vi "CPP-5168-PressureAnalysis-2012.vi"() -> (5 "Plug in titles":string[](array[string]), 7 "Plug in values":string[](array[string]))   [LabVIEW 2012]
uses:
  Globals/Meas_global.vi
  <vilib>/Analysis/baseanly.llb/Mean (DBL).vi
  <vilib>/measure/mascope.llb/Transition Measurements 1 chan.vi
  <vilib>/measure/NI_MAPro.lvlib
  <vilib>/Analysis/NI_AALBase.lvlib
panel:
  out "ValveShutAt":dbl format="%.2f"
  out "SourceOffIndex":i32
  out "nOpen":i32
  out "Zeroes?":bool
  out "Zeroes":dbl[](array[numeric])
  out "Data":dbl[][](array[numeric]) caption="ZeroedCompensatedCalibratedData" format="%#_3g"
  out "ChannelNames":string[](array[string])
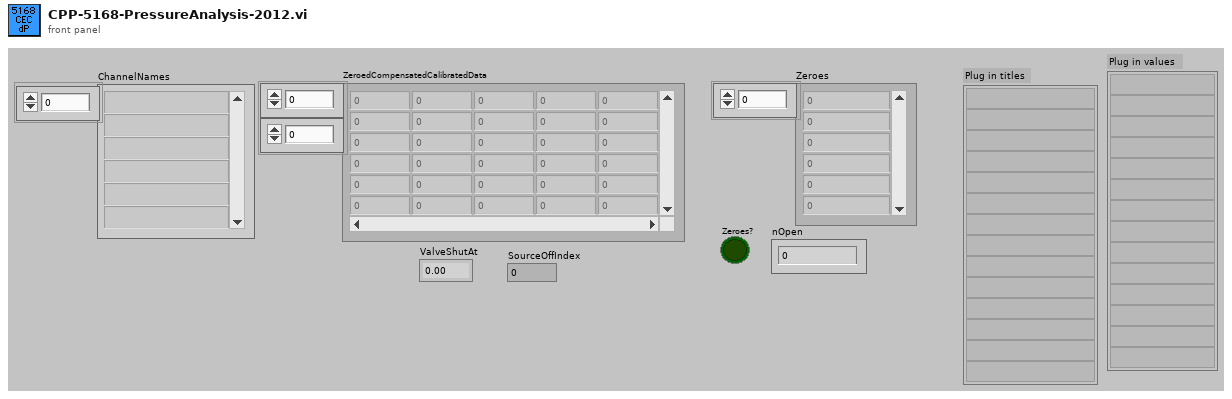
[diagram p1: front panel]
types:
  T1 = typedef "Analysis_info_cluster.ctl" = cluster{"Colour":u32, "Inst type":T2, "Inst name":string, "Symbol":string, "Code name":string, "Extra Info":string, "Inst Array":T3, "Extra Titles":string[], "Extra Values":string[], "U":dbl, "u^2":dbl, "u^3":dbl, "u^4":dbl, "Skew_u":dbl, "Kurt_u":dbl, "Sd Error in Mean":dbl, "% u'/U":dbl, "X":dbl, "Y":dbl, "Z":dbl, "Timescale integral to 25%":dbl, "Sd Error in Variance":dbl, "Calib File":path, "Calib Constants":dbl[], "Output Position":bool, "Full Stats":bool, "Av Sampling Rate":dbl, "Av No of Samples":dbl, "Total Meas Time (s)":dbl, "ADAM Ch Name":string}
  T2 = typedef "Inst_type.ctl" = enum16{"Propeller anemometer", "Raw voltage", "Pressure Transducer", "Pitot-static tube", "Preston tube", "Hot wire", "Cross wire 1", "Cross wire 2", "Generic Linear", "Generic Polynomial", "Generic BackPoly", "Fast FID", "Thermocouple", "Cold wire", "Pulsed Wire", "LDA Vel", "LDA Tran time", "LDA Arr time"}
  T3 = typedef "Instrument_Array.ctl" = enum16{"PWA", "LDA", "Analogue"}
  T4 = typedef "Time_Trace_Cluster.ctl" = cluster{"Weighting":dbl[], "Time (s)":dbl[], "Voltage":dbl[], "Eng Values":dbl[]}
  T5 = cluster{"start time":dbl, "end time":dbl, "ref levels":cluster{"high ref level":dbl, "mid ref level":dbl, "low ref level":dbl, "ref units":u16}}
  T6 = typedef "WindowDescriptor.ctl" = cluster{"Window\nName":string, "SurroundingTaps":string[], "TapWeights":dbl[], "OpenArea\nmm^2":dbl, "OpenArea\nFraction":dbl}
  T7 = typedef "WindowTimeseriesCluster.ctl" = cluster{"Name":string, "OpenArea(mm^2)":dbl, "Timeseries":dbl[]}
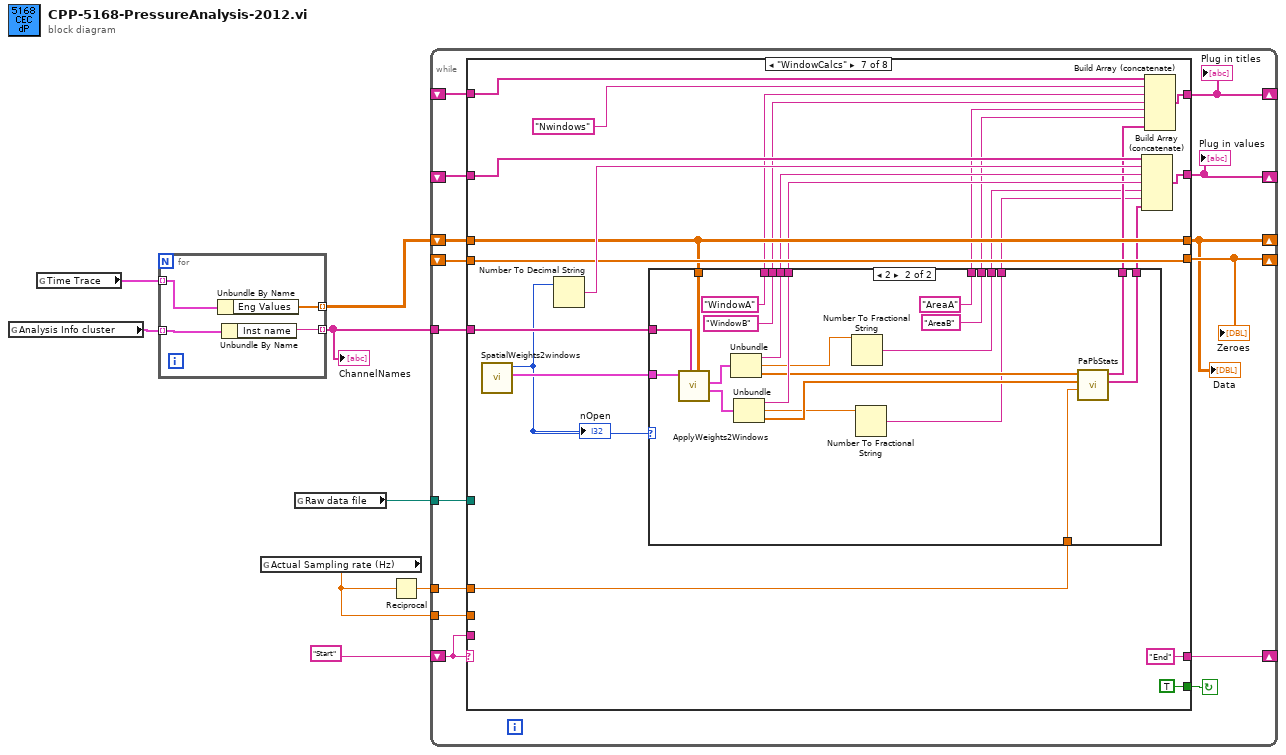
[diagram p0: block diagram]
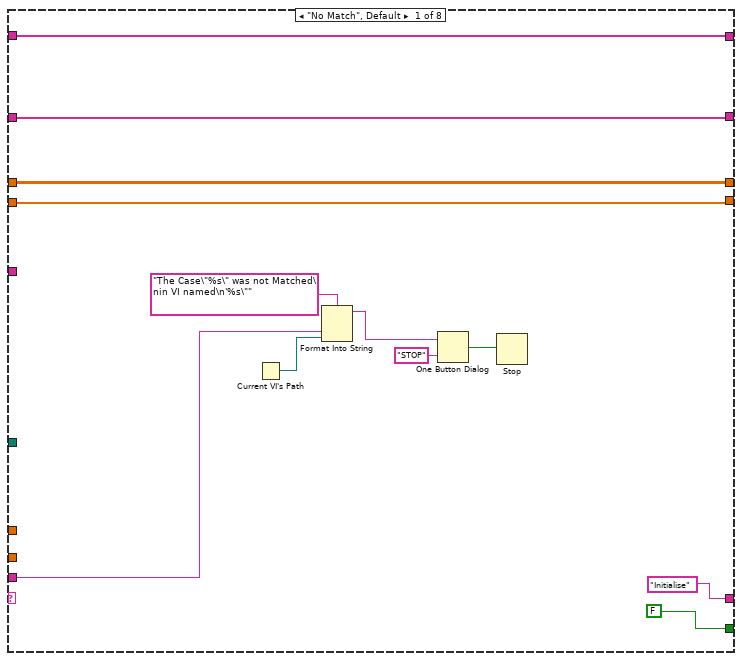
[diagram p2: hidden frame]
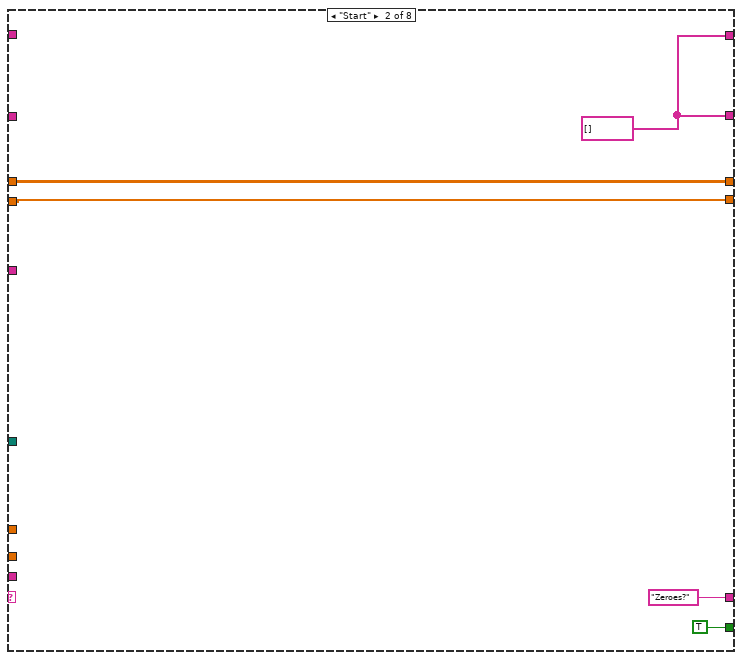
[diagram p3: hidden frame]
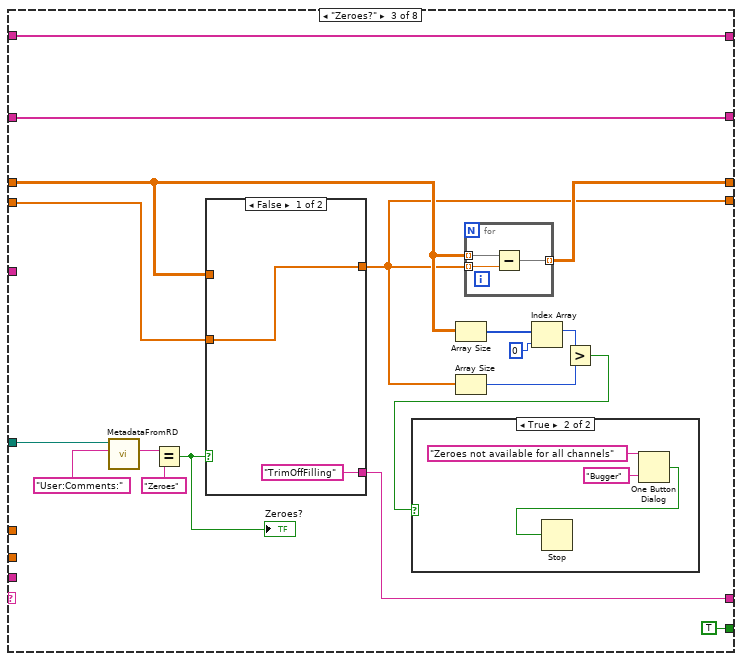
[diagram p4: hidden frame]
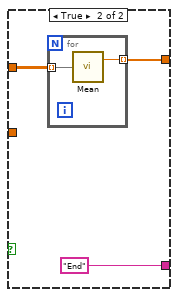
[diagram p6: hidden frame]
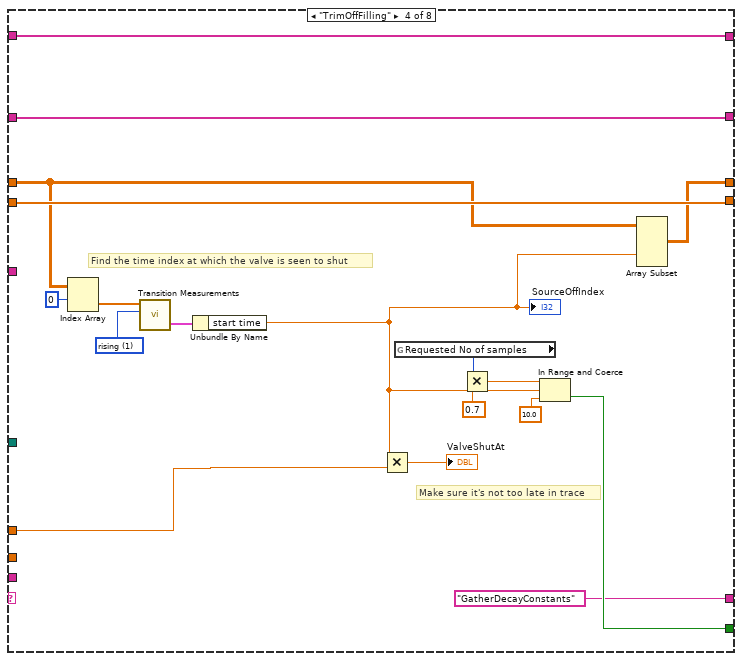
[diagram p7: hidden frame]
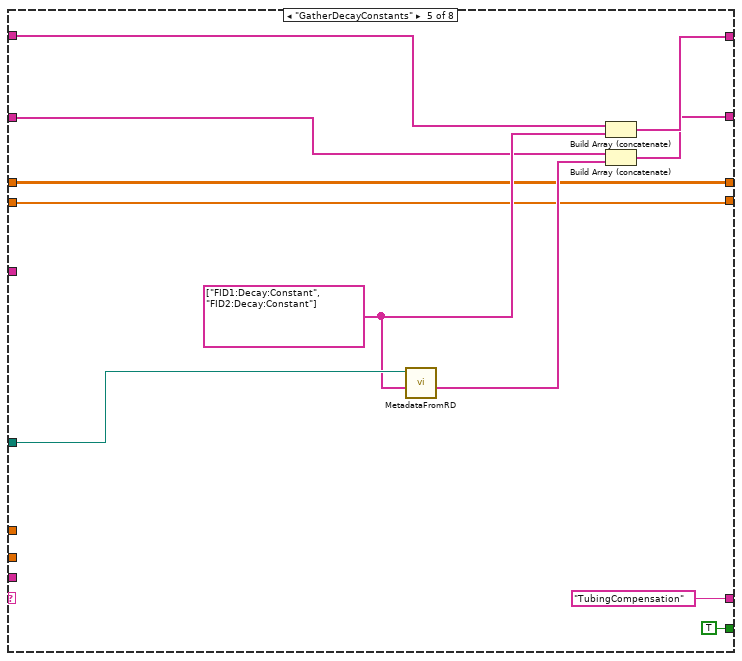
[diagram p8: hidden frame]
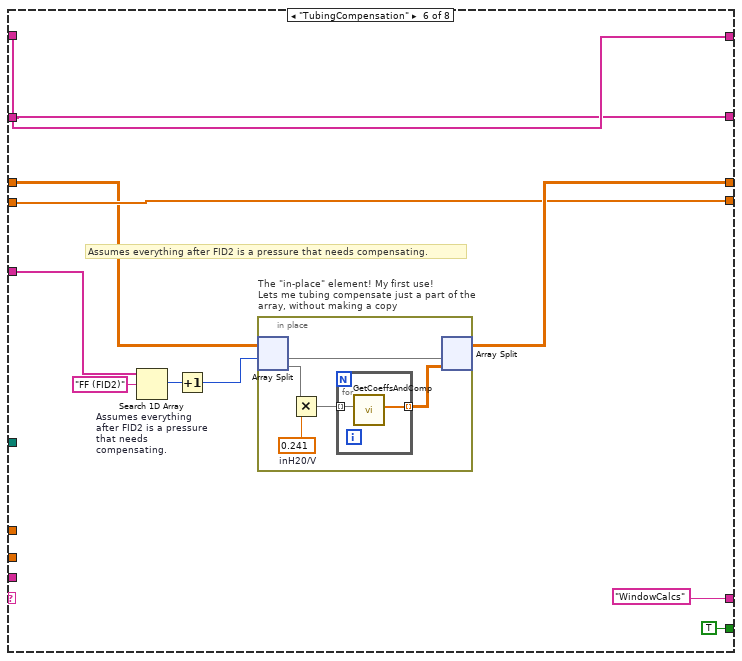
[diagram p9: hidden frame]
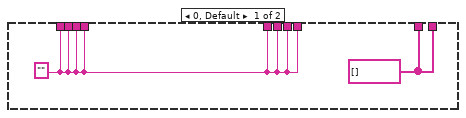
[diagram p10: hidden frame]
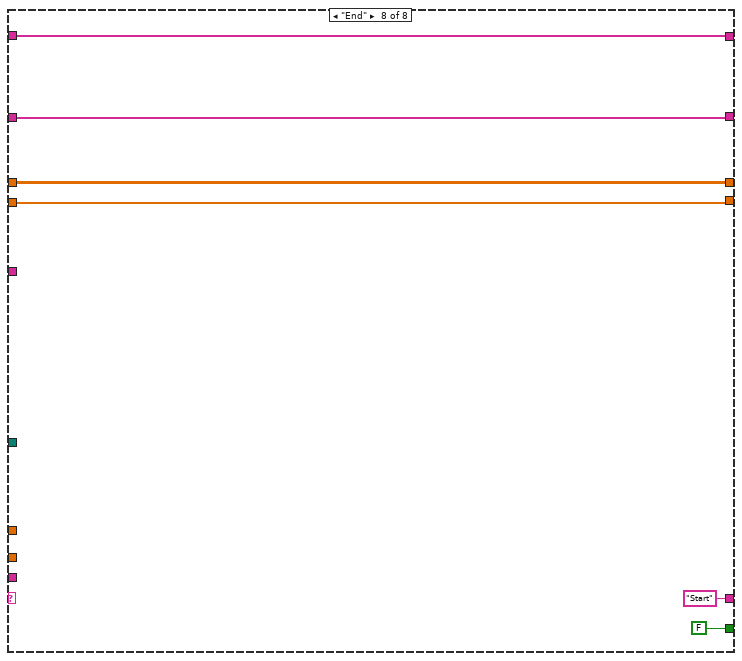
[diagram p11: hidden frame]
diagram:
  n1 = global read "Meas_global.vi" "Analysis Info cluster"() -> (w5:T1[])
  n2 = global read "Meas_global.vi" "Time Trace"() -> (w1:T4[])
  n3 = for {
    tunnel: w5 -> [w12] mode=indexing
    tunnel: [w11] -> w4 mode=indexing
    tunnel: [w9] -> w2 mode=indexing
    tunnel: w1 -> [w10] mode=indexing
    n4 = Unbundle By Name(w10) -> ("Eng Values"=w9:dbl[])
    n5 = Unbundle By Name(w12) -> ("Inst name"=w11:string)
  }
  "ChannelNames" <- w4
  n6 = global read "Meas_global.vi" "Actual Sampling rate (Hz)"() -> (w7:dbl)
  n7 = global read "Meas_global.vi" "Raw data file"() -> (w3:path)
  n8 = Reciprocal(x=w7) -> (1/x=w6:dbl)
  n9 = while {
    shift-left: "Start" -> [w25]
    shift-right: [w26] -> _
    tunnel: w7 -> [w24]
    tunnel: w6 -> [w23]
    tunnel: w4 -> [w21]
    tunnel: w3 -> [w20]
    shift-right: [w14] -> _
    shift-left: _ -> [w19]
    shift-right: [w15] -> _
    shift-left: _ -> [w18]
    shift-right: [w17] -> _
    shift-left: _ -> [w16]
    shift-right: [w13] -> _
    shift-left: w2 -> [w22]
    stop <- w27 continue-if-true
    n10 = case shown="\"WindowCalcs\"" w25 {
      tunnel: [FALSE TRUE ("Processing last block?") TRUE ("Processing last block?") w80 TRUE ("Processing last block?") TRUE ("Processing last block?") TRUE ("Processing last block?") FALSE ("Processing last block?")] -> w27
      tunnel: ["Initialise" "Zeroes?" w53 "GatherDecayConstants" "TubingCompensation" ("f") "WindowCalcs" ("f") "End" ("f") "Start" ("f")] -> w26
      tunnel: w25 -> [w34 _ _ _ _ _ _ _]
      tunnel: w24 -> [_ _ _ _ _ _ _ _]
      tunnel: w23 -> [_ _ _ w81 _ _ w129 _]
      tunnel: w22 -> [w28 w40 w51 w78 w95 w105 w135 w169]
      tunnel: w21 -> [_ _ _ _ _ w110 w139 _]
      tunnel: w20 -> [_ _ w62 _ w103 _ _ _]
      tunnel: w19 -> [w31 _ w60 w93 w100 w108 w142 w172]
      tunnel: [w31 w42 w60 w93 w101 w108 w143 w172] -> w14
      tunnel: [w30 w42 w59 w92 w98 w107 w140 w171] -> w15
      tunnel: w18 -> [w30 _ w59 w92 w97 w107 w141 w171]
      tunnel: [w29 w41 w50 w91 w96 w106 w138 w170] -> w17
      tunnel: w16 -> [w29 w41 w55 w91 w96 w106 w138 w170]
      tunnel: [w28 w40 w52 w77 w95 w109 w135 w169] -> w13
      frame "No Match", Default {
        n11 = Current VI's Path() -> (path=w33:path)
        n12 = Format Into String(format string="The Case\"%s\" was not Matched\nin VI named\n'%s\"" ("Format String"), w34, w33) -> (resulting string=w37:string)  [unwired: 2 in, 1 out]
        n13 = One Button Dialog(message=w37, button name ("OK")="STOP") -> (true=w35:bool)
        n14 = Stop(stop? (T)=w35) -> ()
      }
      frame "Start" {
        w42 = string[] []
      }
      frame "Zeroes?" {
        n15 = call "MetadataFromRD.vi"("ChannelName"="User:Comments:", "Raw data file"=w62) -> ("ValueString"=w57:string)  [unwired: 8 in, 1 out]
        n16 = Equal?(x=w57, y="Zeroes") -> (x = y?=w54:bool)
        "Zeroes?" <- w54
        n17 = case shown="False" w54 {
          tunnel: w51 -> [_ w72]
          tunnel: w55 -> [w69 _]
          tunnel: ["TrimOffFilling" ("f") "End" ("f")] -> w53
          tunnel: [w69 w71] -> w50
          frame False {
          }
          frame True {
            n18 = for {
              tunnel: w72 -> [w75] mode=indexing
              tunnel: [w74] -> w71 mode=indexing
              n19 = call-poly <vilib>:"Mean.vi"("X"=w75) -> ("mean"=w74:dbl)  [unwired: 1 out]
            }
          }
        }
        n20 = Array Size(array=w51) -> (size(s)=w49:i32[])
        n21 = Array Size(array=w50) -> (size(s)=w48:i32)
        n22 = for {
          tunnel: w51 -> [w67] mode=indexing
          tunnel: w50 -> [w68] mode=indexing
          tunnel: [w66] -> w52 mode=indexing
          n23 = Subtract(x=w67, y=w68) -> (x-y=w66:dbl[])
        }
        n24 = Index Array(array=w49, index=0) -> (element=w47:i32)
        n25 = Greater?(x=w47, y=w48) -> (0:w45:bool)
        n26 = case shown="True" w45 {
          frame False {
          }
          frame True {
            n27 = One Button Dialog(message="Zeroes not available for all channels", button name ("OK")="Bugger") -> (true=w63:bool)
            n28 = Stop(stop? (T)=w63) -> ()
          }
        }
      }
      frame "TrimOffFilling" {
        w90 = u16 1 items=["falling", "rising"] ("Valvetransition")
        # "Make sure it's not too late in trace"
        # "Find the time index at which the valve is seen to shut"
        n29 = Index Array(array=w78, index (row)=0) -> (element=w83:dbl[])  [unwired: 1 in]
        n30 = call-poly <vilib>:"Transition Measurements.vi"("polarity (rising)"=w90, "signal in"=w83) -> ("measurement info"=w89:T5)  [unwired: 4 in, 5 out]
        n31 = Unbundle By Name(w89) -> ("start time"=w76:dbl)
        "SourceOffIndex" <- w76
        n32 = Multiply(x=w76, y=w81) -> (x*y=→"ValveShutAt":dbl)
        n33 = global read "Meas_global.vi" "Requested No of samples"() -> (w88:i32)
        n34 = Multiply(x=w88, y=0.7 ("lower limit")) -> (x*y=w86:dbl)
        n35 = In Range and Coerce(upper limit=w86, x=w76, lower limit=10.0) -> (In Range?=w80:bool)  [unwired: 1 out]
        n36 = Array Subset(array=w78, index (col)=w76) -> (w77:dbl[][])  [unwired: 3 in]
      }
      frame "GatherDecayConstants" {
        w102 = string[] ["FID1:Decay:Constant", "FID2:Decay:Constant"] ("Plug in titles")
        n37 = call "MetadataFromRD.vi"("ChannelNames"=w102, "Raw data file"=w103) -> ("ValueStrings"=w99:string[])  [unwired: 8 in, 1 out]
        n38 = Build Array (concatenate)(w100, w102) -> (w101:string[])
        n39 = Build Array (concatenate)(w97, w99) -> (w98:string[])
      }
      frame "TubingCompensation" {
        # "Assumes everything after FID2 is a pressure that needs compensating."
        n40 = Search 1D Array "Assumes everything after FID2 is a pressure that needs compensating."(1D array=w110, element="FF (FID2)") -> (index of element=w112:i32)  [unwired: 1 in]
        n41 = Increment(x=w112) -> (x+1=w111:i32)
        n42 = in-place "The \"in-place\" element! My first use!\nLets me tubing compensate just a part of the array, without making a copy" {
          w116 = 0.241  # inH20/V
          n43 = in-place-split #1(w105, w111) -> (w120:dbl[][], w119:dbl[][])
          n44 = Multiply(x=w119, y=w116) -> (x*y=w117:dbl[][])
          n45 = for {
            tunnel: w117 -> [w122] mode=indexing
            tunnel: [w121] -> w118 mode=indexing
            n46 = call "GetCoeffsAndComp.vi"("mutedData"=w122) -> ("boostedData"=w121:dbl[])  [unwired: 10 in]
          }
          n47 = in-place-split #1(w120, w118) -> (w109:dbl[][])  [unwired: 1 out]
        }
      }
      frame "WindowCalcs" {
        n48 = call "SpatialWeights2windows.vi"() -> ("WindowAveragingInformation"=w144:T6[], "nOpen"=w127:i32)  [unwired: 10 in]
        "nOpen" <- w127
        n49 = Number To Decimal String(number=w127) -> (decimal integer string=w146:string)  [unwired: 1 in]
        n50 = case shown="2" w127 {
          tunnel: w144 -> [_ w168]
          tunnel: w139 -> [_ w167]
          tunnel: w135 -> [_ w166]
          tunnel: [w147 "WindowA" ("element")] -> w134
          tunnel: [w147 "WindowB" ("element")] -> w133
          tunnel: [w147 w161] -> w132
          tunnel: [w147 w160] -> w131
          tunnel: [w148 w159] -> w130
          tunnel: w129 -> [_ w156]
          tunnel: [w148 w155] -> w128
          tunnel: [w147 "AreaA" ("element")] -> w126
          tunnel: [w147 "AreaB" ("element")] -> w125
          tunnel: [w147 w150] -> w124
          tunnel: [w147 w149] -> w123
          frame 0, Default {
            w148 = string[] [] ("Titles")
            w147 = "" ("element")
          }
          frame 2 {
            n51 = call "ApplyWeights2Windows.vi"("ZeroedCompensatedCalibratedData"=w166, "ChannelNames"=w167, "WindowAveragingInformation"=w168) -> ("WindowB"=w164:T7, "WindowA"=w165:T7)  [unwired: 5 in]
            n52 = Unbundle(w165) -> ("Name"=w161:string, "OpenArea(mm^2)"=w153:dbl, "Timeseries"=w158:dbl[])
            n53 = Unbundle(w164) -> ("Name"=w160:string, "OpenArea(mm^2)"=w154:dbl, "Timeseries"=w157:dbl[])
            n54 = Number To Fractional String(number=w153) -> (F-format string=w150:string)  [unwired: 3 in]
            n55 = Number To Fractional String(number=w154) -> (F-format string=w149:string)  [unwired: 3 in]
            n56 = call "PaPbStats.vi"("dT"=w156, "TimeseriesB"=w157, "TimeseriesA"=w158) -> ("Values"=w155:string[], "Titles"=w159:string[])  [unwired: 7 in]
          }
        }
        n57 = Build Array (concatenate)(w141, w146, w132, w131, w124, w123, w128) -> (w140:string[])
        n58 = Build Array (concatenate)(w142, "Nwindows", w134, w133, w126, w125, w130) -> (w143:string[])
      }
      frame "End" {
      }
    }
    "Plug in values" <- w15
    "Plug in titles" <- w14
    "Data" <- w13
    "Zeroes" <- w17
  }
